vi "Z2BendTwist.vi"(8 "Twist offset [V]":fxp<+/-,26,4>, 9 "Bend offset [V]":fxp<+/-,26,4>, 10 "Hall3 [V]":fxp<+,25,3>, 11 "Hall2 [V]":fxp<+,25,3>) -> (2 "Twist [V]":fxp<+/-,25,4>, 3 "Bend [V]":fxp<+/-,25,4>)   [LabVIEW 2017, in "FPGA functions.lvlib"]
doc: "Convert z measurments into bend and twist"
uses:
  FPGA functions.lvlib
  <vilib>/Platform/TimedLoop/XDataNode/XDataNode.xnode
  <vilib>/Platform/TimedLoop/XDataNode/nitl_modes.ctl
  <vilib>/Platform/TimedLoop/XDataNode/XDNodeRunTimeDep.lvlib
  <vilib>/Platform/TimedLoop/XDataNode/wakeup.ctl
  <vilib>/Platform/TimedLoop/XDataNode/timing_clust.ctl
  <vilib>/rvi/FXPMathLib/FxpAdd/XNode/nifxpmath_Add.xnode
  <vilib>/rvi/FXPMathLib/FxpSub/XNode/nifxpmath_Sub.xnode
  <vilib>/rvi/FXPMathLib/sim/FxpSim.dll
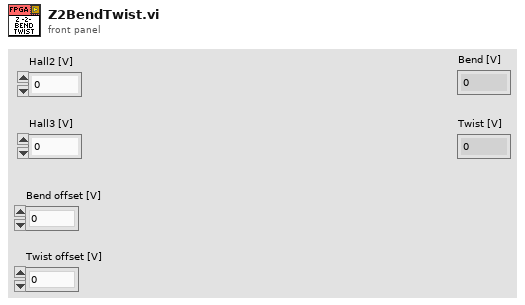
[diagram p1: front panel]
types:
  T1 = typedef "XDNodeRunTimeDep.lvlib/timing_clust.ctl" = cluster{"Expected End [f-1]":u64, "Actual End [f-1]":u64, "Finished Late? [f-1]":bool, "Expected End [i-1]":u64, "Actual End [i-1]":u64, "Finished Late? [i-1]":bool, "Expected Start [i]":u64, "Actual Start [i]":u64, "Expected Start [f]":u64, "Actual Start [f]":u64, "Source Name":string, "Structure Name":string, "Period":i64, "Deadline":i64, "Offset":i64, "Start":i64, "Priority":i32, "Timeout":i32, "Mode":T2, "Wakeup Reason":T3, "Error":errorcluster, "Source Type":string, "Secondary Source Type":string, "Global End Time":u64, "Global Start Time":u64, "Frame Duration":u64, "Iteration Duration":u64, "Assigned CPU":i32, "I/O Scan Engine Mode":u32}
  T2 = typedef "XDNodeRunTimeDep.lvlib/nitl_modes.ctl" = enum32{"No Change", "Process missed periods, maintain original phase", "Discard missed periods, maintain original phase", "Process missed periods, ignore original phase", "Discard missed periods, ignore original phase"}
  T3 = typedef "XDNodeRunTimeDep.lvlib/wakeup.ctl" = enum32{"Normal", "Aborted", "Asynchronous wakeup", "Timing source error", "Timed loop error", "Timeout"}
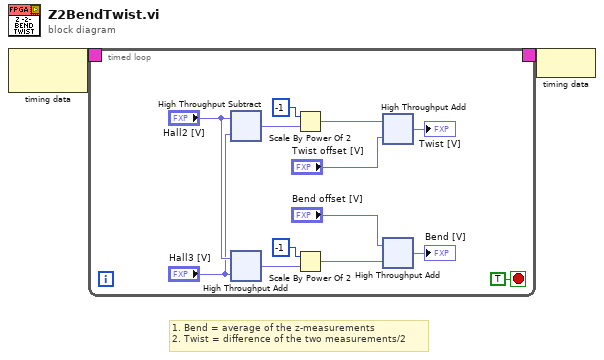
[diagram p0: block diagram]
diagram:
  # "1. Bend = average of the z-measurements\n2. Twist = difference of the two measurements/2"
  n1 = node-c288() -> (w2:T1)  [unwired: 1 in]
  n2 = timed-loop {
    timing: w2 -> [_]
    timing-out: [_] -> w1
    stop <- TRUE stop-if-true
    n3 = xnode ("High Throughput Subtract")("x"="Hall2 [V]", "y"="Hall3 [V]") -> ("x-y"=w9:fxp<+/-,27,4>)
    n4 = xnode ("High Throughput Add")("x"="Hall2 [V]", "y"="Hall3 [V]") -> ("x+y"=w14:fxp<+,27,4>)
    n5 = Scale By Power Of 2(n=i16 -1, x=w9) -> (x*2^n=w3:fxp<+/-,27,4>)
    n6 = Scale By Power Of 2(n=i16 -1, x=w14) -> (x*2^n=w4:fxp<+,27,4>)
    n7 = xnode ("High Throughput Add")("x"=w3, "y"="Twist offset [V]") -> ("x+y"=→"Twist [V]":fxp<+/-,25,4>)
    n8 = xnode ("High Throughput Add")("x"="Bend offset [V]", "y"=w4) -> ("x+y"=→"Bend [V]":fxp<+/-,25,4>)
  }
  n9 = node-c288(w1) -> ()
